vi "read default value Array of Boolean.vi"(8 "error in":errorcluster, 11 "system tag in":refnum<class "tag descriptor.lvclass">) -> (0 "error out":errorcluster, 1 "invalid":bool, 2 "default value":bool[](array[boolean]), 3 "system tag out":refnum<class "tag descriptor.lvclass">)   [LabVIEW 2013, in "tag bus.lvlib" / "tag descriptor.lvclass"]
doc: "Converts the raw default value stored in the tag to the type specified by the polymorph."
uses:
  tag descriptor.lvclass
  Data Type.ctl
  tag descriptor.lvclass/tag descriptor.ctl
  tag bus.lvlib
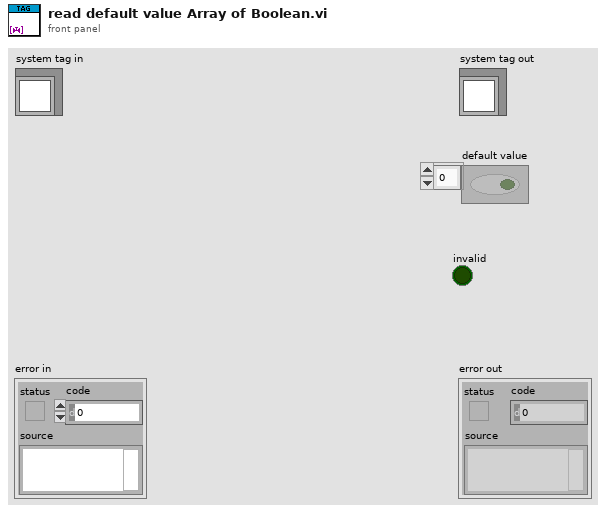
[diagram p1: front panel]
types:
  T1 = typedef "tag bus.lvlib/tag descriptor.lvclass/Data Type.ctl" = enum16{"Double", "Single", "I64", "I32", "I16", "I8", "U64", "U32", "U16", "U8", "Boolean", "String", "Array of Double", "Array of Single", "Array of I64", "Array of I32", "Array of I16", "Array of I8", "Array of U64", "Array of U32", "Array of U16", "Array of U8", "Array of Boolean", "Array of String"}
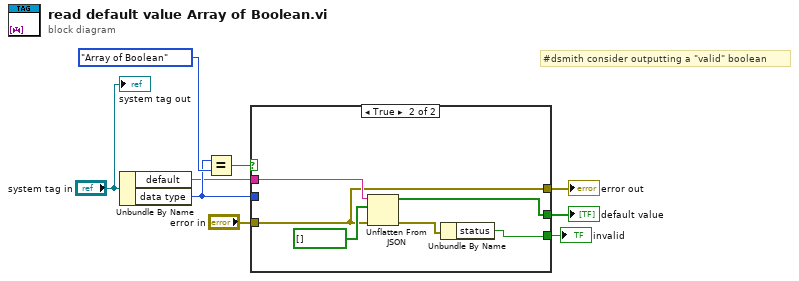
[diagram p0: block diagram]
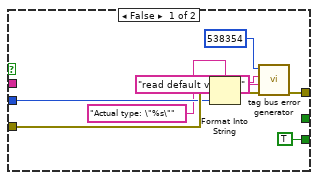
[diagram p2: hidden frame]
diagram:
  # "#dsmith consider outputting a \"valid\" boolean"
  n1 = Unbundle By Name("system tag in") -> ("default"=w3:string, "data type"=w4:T1)
  n2 = Equal?(x=w4, y=Data_Type."Array of Boolean") -> (x = y?=w7:bool)
  n3 = case shown="True" w7 {
    tunnel: "error in" -> [w18 w22]
    tunnel: [w14 w22] -> w5
    tunnel: w4 -> [w13 _]
    tunnel: w3 -> [_ w23]
    tunnel: [_ w21] -> w2
    tunnel: [TRUE ("status") w19] -> w1
    frame False {
      n4 = Format Into String(format string="Actual type: \"%s\"", error in=w18, w13) -> (resulting string=w15:string, error out=w16:errorcluster)  [unwired: 1 in]
      n5 = call "tag bus error generator.vi"("error in"=w16, "source"="read default value.vi", "append error message"=w15, "error code (0)"=538354) -> ("error out"=w14:errorcluster)  [unwired: 5 in]
    }
    frame True {
      n6 = Unflatten From JSON(JSON string=w23, type and defaults=bool[] [] ("default value"), error in (no error)=w22) -> (value=w21:bool[], error out=w20:errorcluster)  [unwired: 4 in]
      n7 = Unbundle By Name(w20) -> ("status"=w19:bool)
    }
  }
  "error out" <- w5
  "default value" <- w2
  "invalid" <- w1
  "system tag out" <- "system tag in"
